vi "Obis Control.vi"(0 "Laser Notifier Element":T1={"Laser Action"=enum."Set On/Off", "Received?"=FALSE, "Enabled (Interlock)?"=FALSE, "Light Emission?"=FALSE, "Power (mW)"=0.0, "Settings"={"Laser Parameters"=enum."Wavelength (nm)", "Value"=0.0}, "Status"=enum."Error", "Error"={"status"=FALSE, "code"=0, "source"=""}}, 11 "VISA Ref":refnum<visa-resource-name>) -> (4 "Laser Notifier Element":T1={"Laser Action"=enum."Set On/Off", "Received?"=FALSE, "Enabled (Interlock)?"=FALSE, "Light Emission?"=FALSE, "Power (mW)"=0.0, "Settings"={"Laser Parameters"=enum."Wavelength (nm)", "Value"=0.0}, "Status"=enum."Error", "Error"={"status"=FALSE, "code"=0, "source"=""}})   [LabVIEW 2020]
uses:
  Laser Controls/Laser Notifier Element.ctl
  Laser Controls/Laser Actions.ctl
  Laser Controls/Laser Settings.ctl
  Laser Controls/Laser Parameters.ctl
  Laser Controls/Laser Status.ctl
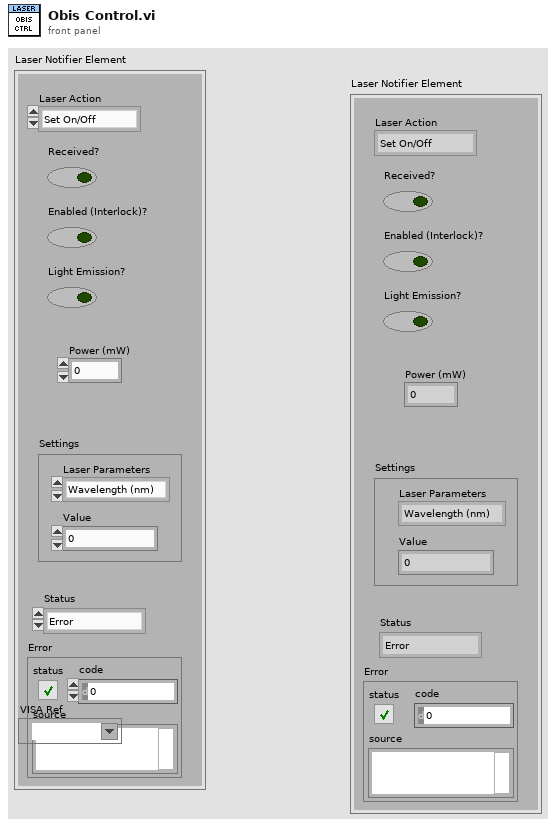
[diagram p1: front panel]
types:
  T1 = typedef "Laser Notifier Element.ctl" = cluster{"Laser Action":T2, "Received?":bool, "Enabled (Interlock)?":bool, "Light Emission?":bool, "Power (mW)":dbl, "Settings":T3, "Status":T5, "Error":errorcluster}
  T2 = typedef "Laser Actions.ctl" = enum16{"Error Check", "Set On/Off", "Set Power", "Set Parameter", "Get Power", "Get Status", "Get Parameter", "Quit"}
  T3 = typedef "Laser Settings.ctl" = cluster{"Laser Parameters":T4, "Value":dbl}
  T4 = typedef "Laser Parameters.ctl" = enum16{"Wavelength (nm)", "Pulsing?", "Rep. Rate", "External Control"}
  T5 = typedef "Laser Status.ctl" = enum16{"Warmup", "Ready", "Emission", "Tuning", "Error"}
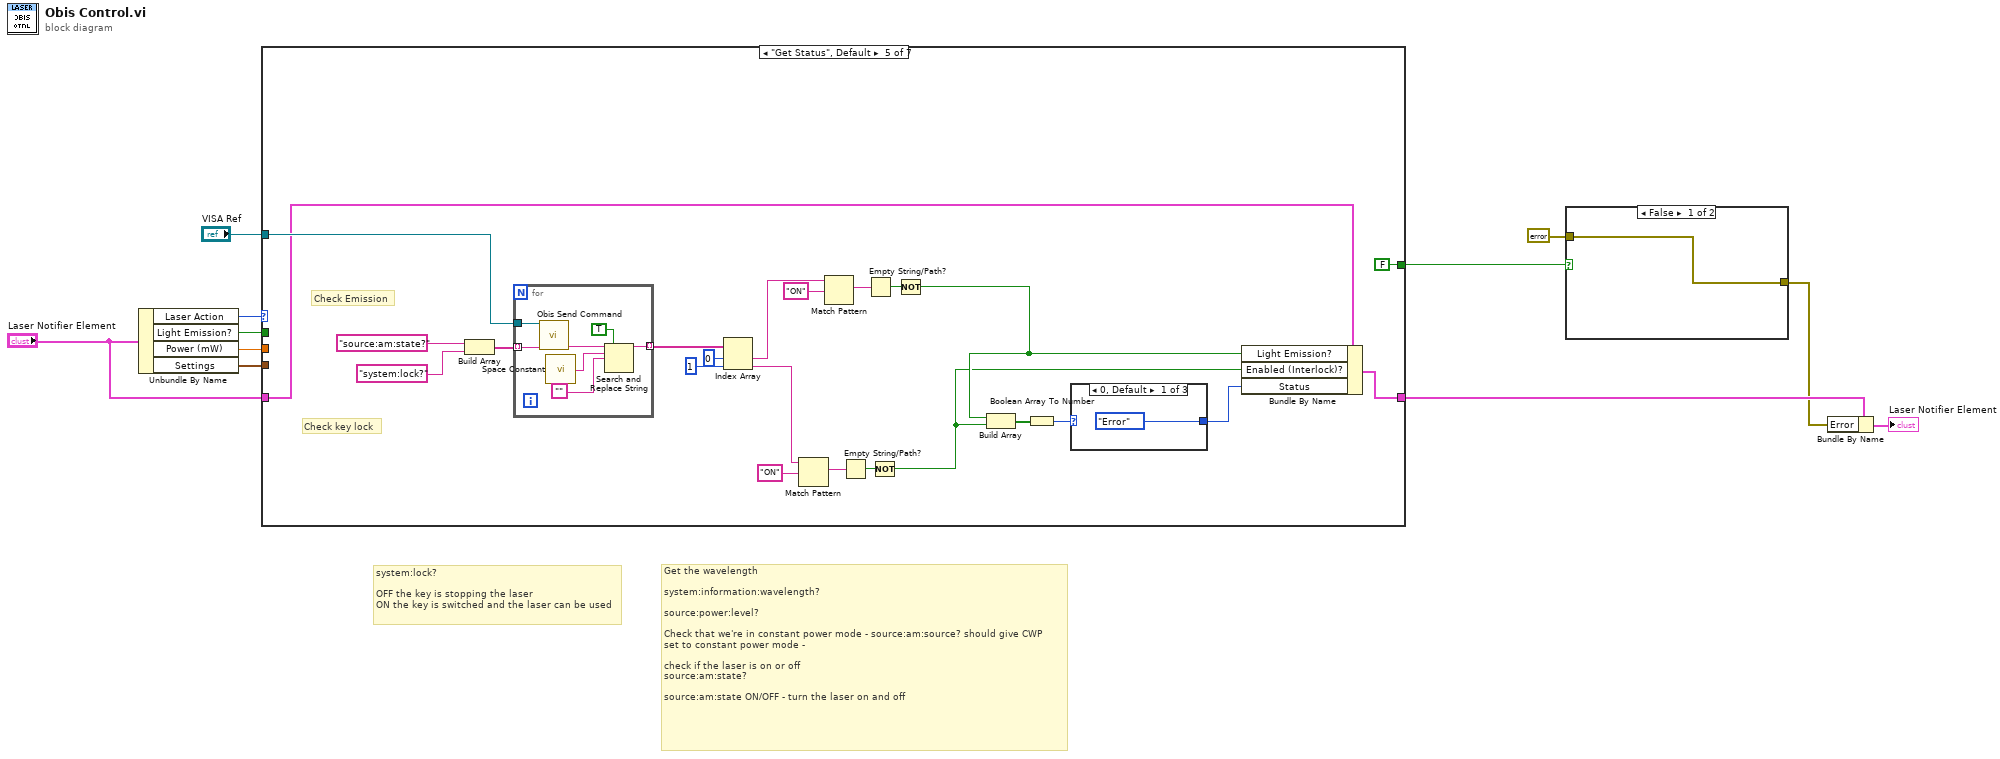
[diagram p0: block diagram]
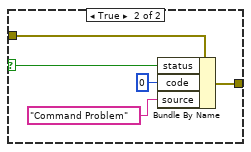
[diagram p2: hidden frame]
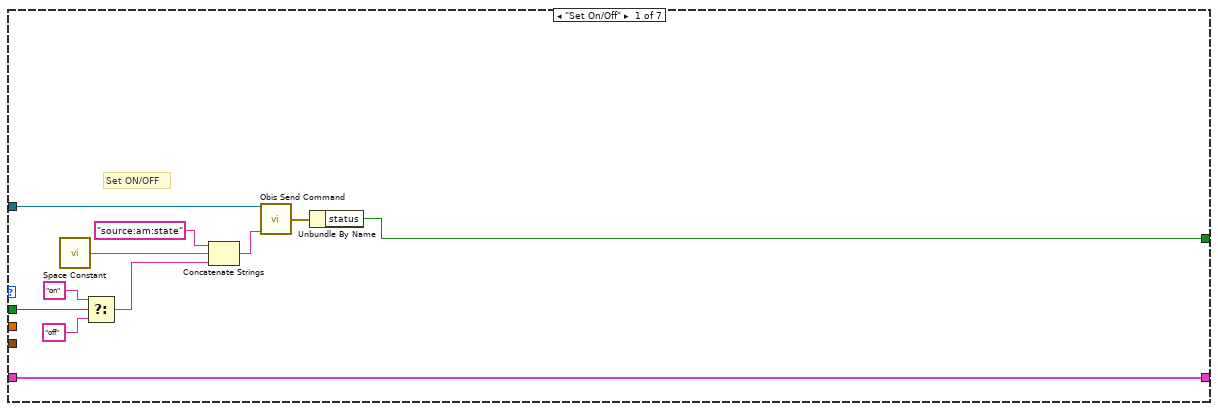
[diagram p3: hidden frame]
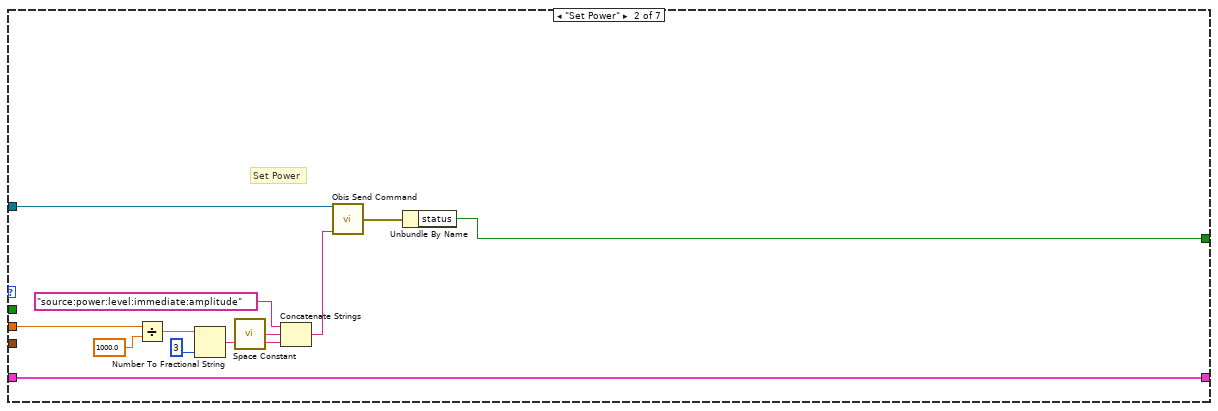
[diagram p4: hidden frame]
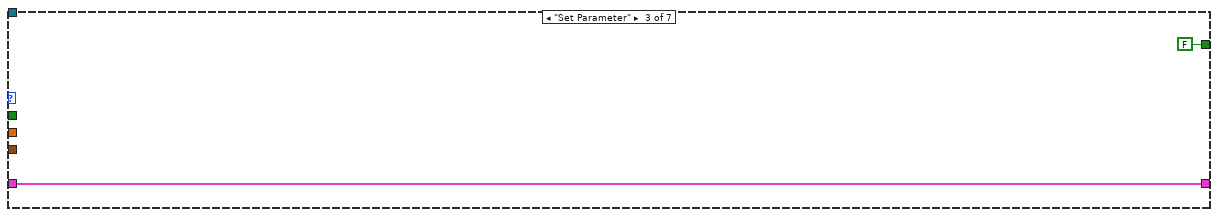
[diagram p5: hidden frame]
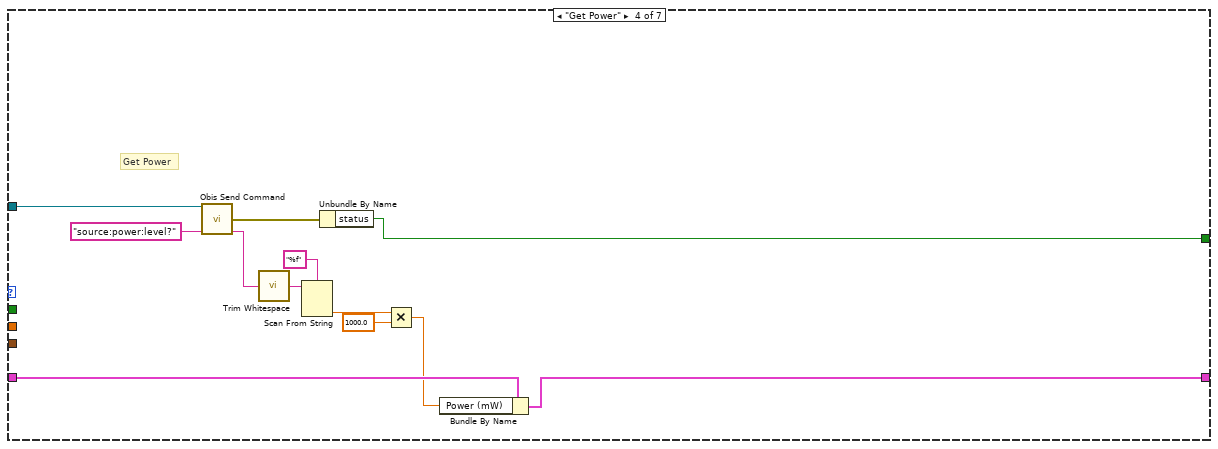
[diagram p6: hidden frame]
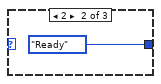
[diagram p7: hidden frame]
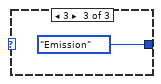
[diagram p8: hidden frame]
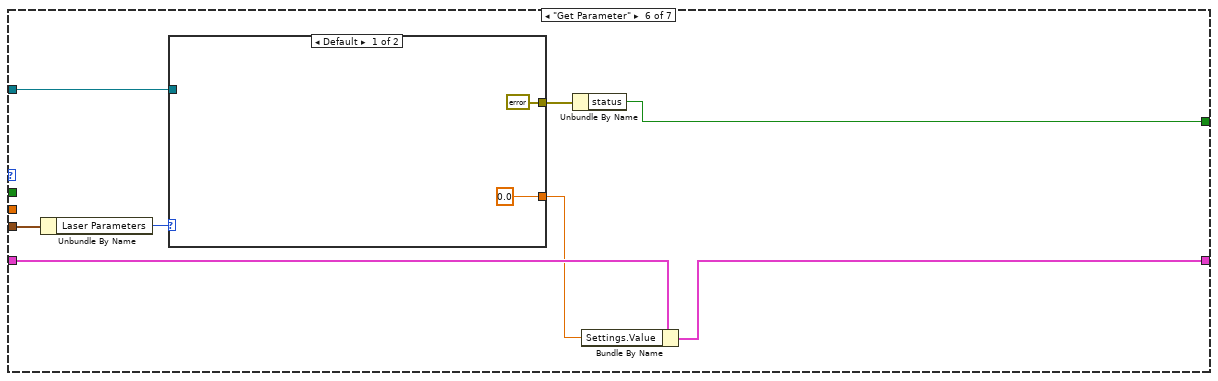
[diagram p9: hidden frame]
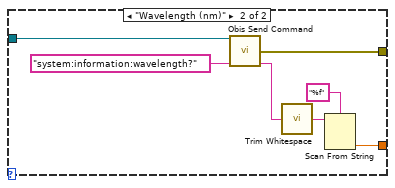
[diagram p10: hidden frame]
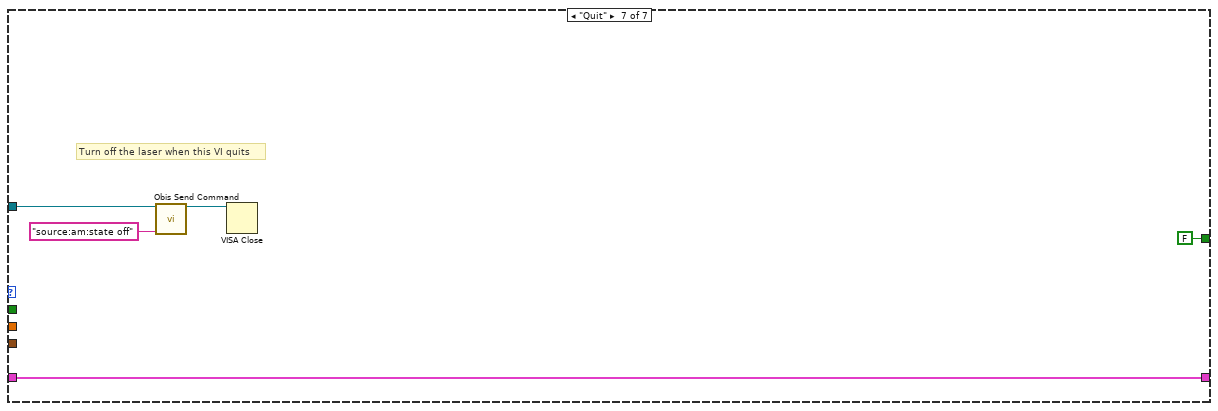
[diagram p11: hidden frame]
diagram:
  # "Get the wavelength\n\nsystem:information:wavelength?\n\nsource:power:level?\n\nCheck that we're in constant power mode - source:am:source? should give CWP\nset to constant power mode -\n\ncheck if the laser is on or off\nsource:am:state?\n\nsource:am:state ON/OFF - turn the laser on and off"
  # "system:lock?\n\nOFF the key is stopping the laser\nON the key is switched and the laser can be used"
  n1 = Unbundle By Name("Laser Notifier Element") -> ("Laser Action"=w11:T2, "Light Emission?"=w5:bool, "Power (mW)"=w4:dbl, "Settings"=w3:T3)
  n2 = case shown="\"Get Status\", Default" w11 {
    tunnel: "VISA Ref" -> [w19 w31 _ w46 w69 w87 w102]
    tunnel: [w18 w30 w36 w44 w68 w84 w101] -> w8
    tunnel: w5 -> [w17 _ _ _ _ _ _]
    tunnel: w4 -> [_ w26 _ _ _ _ _]
    tunnel: w3 -> [_ _ _ _ _ w89 _]
    tunnel: "Laser Notifier Element" -> [w18 w30 w36 w45 w63 w86 w101]
    tunnel: [w12 w23 FALSE ("status") w37 FALSE ("status") w82 FALSE ("status")] -> w1
    frame "Set On/Off" {
      # "Set ON/OFF"
      n3 = call <vilib>:"Space Constant.vi"() -> ("String"=w20:string)
      n4 = Select(t="on", s=w17, f="off") -> (s? t:f=w16:string)
      n5 = Concatenate Strings("source:am:state" ("string"), w20, w16) -> (w22:string)
      n6 = call "Obis Send Command.vi"("VISA Ref"=w19, "Command"=w22) -> ("Error Out"=w13:errorcluster)  [unwired: 11 in, 2 out]
      n7 = Unbundle By Name(w13) -> ("status"=w12:bool)
    }
    frame "Set Power" {
      # "Set Power"
      n8 = Divide(x=w26, y=1000.0) -> (x/y=w25:dbl)
      n9 = Number To Fractional String(number=w25, precision (6)=i16 3) -> (F-format string=w29:string)  [unwired: 2 in]
      n10 = call <vilib>:"Space Constant.vi"() -> ("String"=w28:string)
      n11 = Concatenate Strings("source:power:level:immediate:amplitude" ("string"), w28, w29) -> (w32:string)
      n12 = call "Obis Send Command.vi"("VISA Ref"=w31, "Command"=w32) -> ("Error Out"=w24:errorcluster)  [unwired: 11 in, 2 out]
      n13 = Unbundle By Name(w24) -> ("status"=w23:bool)
    }
    frame "Set Parameter" {
    }
    frame "Get Power" {
      # "Get Power"
      n14 = call "Obis Send Command.vi"("VISA Ref"=w46, "Command"="source:power:level?") -> ("Error Out"=w38:errorcluster, "Response"=w43:string)  [unwired: 11 in, 1 out]
      n15 = call <vilib>:"Trim Whitespace.vi"("string"=w43) -> ("trimmed string"=w47:string)  [unwired: 1 in]
      n16 = Scan From String(format string="%f", input string=w47) -> (output 1=w41:dbl)  [unwired: 3 in, 3 out]
      n17 = Unbundle By Name(w38) -> ("status"=w37:bool)
      n18 = Multiply(x=w41, y=1000.0) -> (x*y=w39:dbl)
      n19 = Bundle By Name(cluster=w45, "Power (mW)"=w39) -> (w44:T1)
    }
    frame "Get Status", Default {
      # "Check Emission"
      # "Check key lock"
      n20 = Build Array("source:am:state?" ("string"), "system:lock?" ("string")) -> (w71:string[])
      n21 = for {
        tunnel: w71 -> [w76] mode=indexing
        tunnel: [w77] -> w66 mode=indexing
        tunnel: w69 -> [w81]
        n22 = call "Obis Send Command.vi"("VISA Ref"=w81, "Command"=w76) -> ("Response"=w75:string)  [unwired: 11 in, 2 out]
        n23 = call <vilib>:"Space Constant.vi"() -> ("String"=w79:string)
        n24 = Search and Replace String(replace all?=TRUE ("replace all? (F)"), input string=w75, search string=w79, replace string="") -> (result string=w77:string)  [unwired: 4 in, 3 out]
      }
      n25 = Index Array(array=w66, index #1=0 ("index"), index #2=1 ("index")) -> (element #1=w56:string, element #2=w50:string)
      n26 = Match Pattern(string=w50, regular expression="ON") -> (match substring=w52:string)  [unwired: 1 in, 3 out]
      n27 = Match Pattern(string=w56, regular expression="ON") -> (match substring=w58:string)  [unwired: 1 in, 3 out]
      n28 = Empty String/Path?(string/path=w52) -> (empty?=w51:bool)
      n29 = Empty String/Path?(string/path=w58) -> (empty?=w55:bool)
      n30 = Not(x=w51) -> (.not. x?=w49:bool)
      n31 = Not(x=w55) -> (.not. x?=w54:bool)
      n32 = Build Array(w54, w49) -> (w62:bool[])
      n33 = Boolean Array To Number(Boolean array=w62) -> (number=w61:u32)
      n34 = case shown="0, Default" w61 {
        tunnel: [Laser_Status."Error" ("Status") Laser_Status."Ready" ("Status") Laser_Status."Emission" ("Status")] -> w60
        frame 0, Default {
        }
        frame 2 {
        }
        frame 3 {
        }
      }
      n35 = Bundle By Name(cluster=w63, "Light Emission?"=w54, "Enabled (Interlock)?"=w49, "Status"=w60) -> (w68:T1)
    }
    frame "Get Parameter" {
      n36 = Unbundle By Name(w89) -> ("Laser Parameters"=w88:T4)
      n37 = case shown="Default" w88 {
        tunnel: w87 -> [_ w98]
        tunnel: [0.0 w93] -> w85
        tunnel: [errorcluster {"status"=FALSE, "code"=0, "source"=""} ("Error Out") w92] -> w83
        frame Default {
        }
        frame "Wavelength (nm)" {
          n38 = call "Obis Send Command.vi"("VISA Ref"=w98, "Command"="system:information:wavelength?" ("Response")) -> ("Error Out"=w92:errorcluster, "Response"=w94:string)  [unwired: 11 in, 1 out]
          n39 = call <vilib>:"Trim Whitespace.vi"("string"=w94) -> ("trimmed string"=w95:string)  [unwired: 1 in]
          n40 = Scan From String(format string="%f", input string=w95) -> (output 1=w93:dbl)  [unwired: 3 in, 3 out]
        }
      }
      n41 = Unbundle By Name(w83) -> ("status"=w82:bool)
      n42 = Bundle By Name(cluster=w86, "Settings.Value"=w85) -> (w84:T1)
    }
    frame "Quit" {
      # "Turn off the laser when this VI quits"
      n43 = call "Obis Send Command.vi"("VISA Ref"=w102, "Command"="source:am:state off") -> ("VISA Ref Out"=w103:refnum<visa-resource-name>)  [unwired: 11 in, 2 out]
      n44 = VISA Close(VISA resource name=w103) -> ()  [unwired: 1 in, 1 out]
    }
  }
  n45 = case shown="False" w1 {
    selector: w1 -> [_ w106]
    tunnel: errorcluster {"status"=FALSE, "code"=0, "source"=""} ("Error") -> [w104 w107]
    tunnel: [w104 w105] -> w6
    frame False {
    }
    frame True {
      n46 = Bundle By Name(cluster=w107, "status"=w106, "code"=0, "source"="Command Problem") -> (w105:errorcluster)
    }
  }
  n47 = Bundle By Name(cluster=w8, "Error"=w6) -> (→"Laser Notifier Element":T1)
